vi "Lock Test VI.vi"(8 "error in (no error)":errorcluster, 9 "Instrument Names":string[](array[string]), 10 "milliseconds to wait":u32, 11 "Sequence Context":refnum<k7>) -> (0 "error out":errorcluster)   [LabVIEW 2019]
uses:
  Lock Step/Lock Library.lvlib
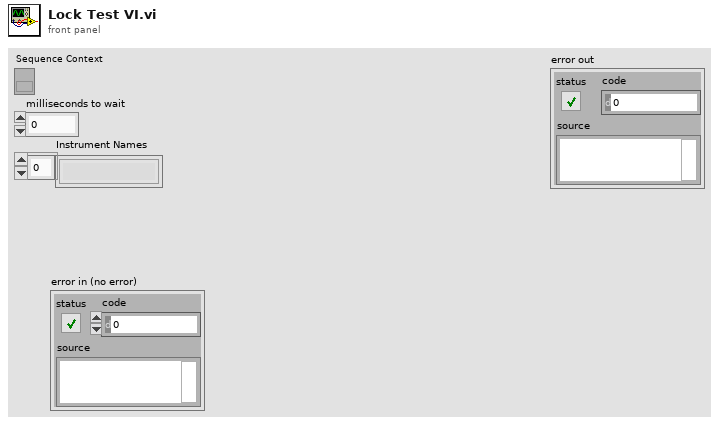
[diagram p1: front panel]
types:
  T1 = typedef "Lock Library.lvlib/References.ctl" = cluster{"Sequence Context":refnum<k7>, "Created Mutexes":refnum<k7>[], "Auto-Release Refs":refnum<k7>[], "SyncManagerRefs":refnum<k7>[], "AutoUnlock?":bool}
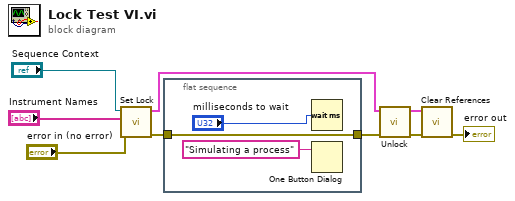
[diagram p0: block diagram]
diagram:
  n1 = call "Set Lock.vi"("error in (no error)"="error in (no error)", "Instrument Names"="Instrument Names", "Sequence Context"="Sequence Context") -> ("error out"=w6:errorcluster, "References"=w8:T1)  [unwired: 6 in, 1 out]
  n2 = flat-sequence {
    tunnel: [w12] -> w7
    tunnel: w6 -> [w12]
    frame #0 {
      n3 = Wait (ms)(milliseconds to wait="milliseconds to wait") -> ()  [unwired: 1 out]
      n4 = One Button Dialog(message="Simulating a process") -> ()  [unwired: 1 in, 1 out]
    }
  }
  n5 = call "Unlock.vi"("error in (no error)"=w7, "References"=w8) -> ("error out"=w5:errorcluster, "References Out"=w2:T1)  [unwired: 8 in]
  n6 = call "Clear References.vi"("error in (no error)"=w5, "References"=w2) -> ("error out"=→"error out":errorcluster)  [unwired: 9 in]
